vi "Lidar Parsing.vi"() -> ()   [LabVIEW 2016]
uses:
  <vilib>/Platform/TimedLoop/XDataNode/timing_clust.ctl
  <vilib>/Platform/TimedLoop/XDataNode/nitl_modes.ctl
  <vilib>/Platform/TimedLoop/XDataNode/wakeup.ctl
  <vilib>/Platform/TimedLoop/XDataNode/XDataNode.xnode
  <vilib>/Platform/TimedLoop/XDataNode/XDNodeRunTimeDep.lvlib
panel:
  out "쉬프트":cluster{dbl[], dbl[]}(graph)
  in  "쉬프트(mm)":dbl=420.0
  in  "Angular resolution 0.25 / 0.5":dbl=0.25
  in  "finish angle":dbl=180.0
  in  "start angle":dbl
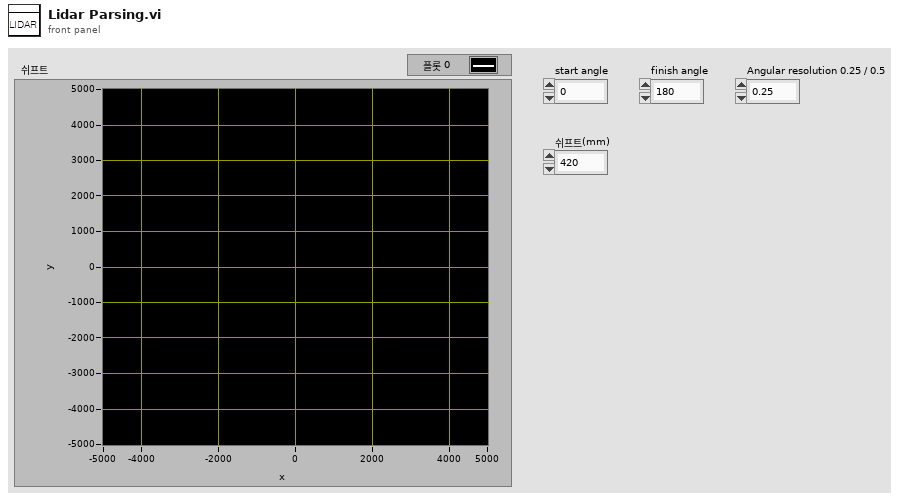
[diagram p1: front panel]
types:
  T1 = enum16{"Standard", "Buffered", "CRLF", "Immediate"}
  T2 = typedef "XDNodeRunTimeDep.lvlib/timing_clust.ctl" = cluster{"Expected End [f-1]":u64, "Actual End [f-1]":u64, "Finished Late? [f-1]":bool, "Expected End [i-1]":u64, "Actual End [i-1]":u64, "Finished Late? [i-1]":bool, "Expected Start [i]":u64, "Actual Start [i]":u64, "Expected Start [f]":u64, "Actual Start [f]":u64, "Source Name":string, "Structure Name":string, "Period":i64, "Deadline":i64, "Offset":i64, "Start":i64, "Priority":i32, "Timeout":i32, "Mode":T3, "Wakeup Reason":T4, "Error":errorcluster, "Source Type":string, "Secondary Source Type":string, "Global End Time":u64, "Global Start Time":u64, "Frame Duration":u64, "Iteration Duration":u64, "Assigned CPU":i32, "I/O Scan Engine Mode":u32}
  T3 = typedef "XDNodeRunTimeDep.lvlib/nitl_modes.ctl" = enum32{"No Change", "Process missed periods, maintain original phase", "Discard missed periods, maintain original phase", "Process missed periods, ignore original phase", "Discard missed periods, ignore original phase"}
  T4 = typedef "XDNodeRunTimeDep.lvlib/wakeup.ctl" = enum32{"Normal", "Aborted", "Asynchronous wakeup", "Timing source error", "Timed loop error", "Timeout"}
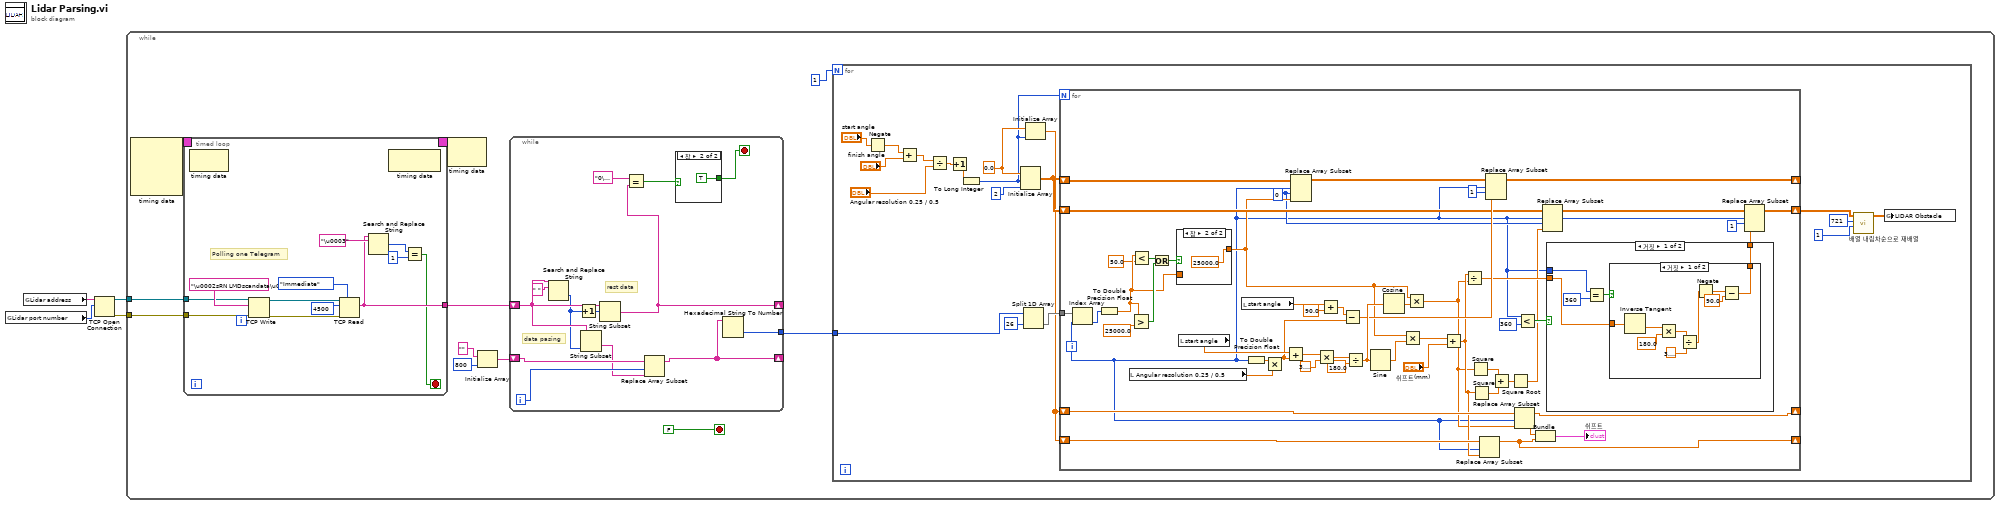
[diagram p0: block diagram]
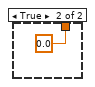
[diagram p2: hidden frame]
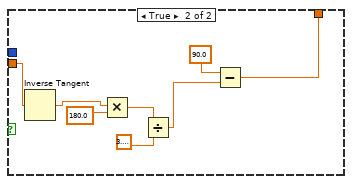
[diagram p3: hidden frame]
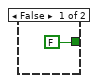
[diagram p5: hidden frame]
diagram:
  n1 = global read "[GV]_LIDAR Port NUM.vi" "Lidar port number"() -> (w1:u16)
  n2 = global read "[GV]_LIDAR Ethernet Address.vi" "Lidar address"() -> (w2:string)
  n3 = TCP Open Connection(address=w2, remote port or service name=w1) -> (connection ID=w4:refnum<k5>, error out=w3:errorcluster)  [unwired: 3 in]
  n4 = while {
    tunnel: w4 -> [w14]
    tunnel: w3 -> [w13]
    stop <- FALSE stop-if-true
    n5 = node-c288() -> (w6:T2)  [unwired: 4 in]
    n6 = timed-loop {
      tunnel: w14 -> [w24]
      tunnel: w13 -> [w23]
      tunnel: [w17] -> w12
      timing: w6 -> [_]
      timing-out: [_] -> w5
      stop <- w16 stop-if-true
      # "Polling one Telegram"
      n7 = node-c288() -> ()  [unwired: 1 in, 1 out]
      n8 = TCP Write(connection ID=w24, data in="\u0002sRN LMDscandata\u0003" ("데이터 입력"), error in (no error)=w23) -> (connection ID out=w27:refnum<k5>, error out=w26:errorcluster)  [unwired: 1 in, 1 out]
      n9 = TCP Read(connection ID=w27, bytes to read=4500 ("읽을 바이트"), error in (no error)=w26, 7:T1."Immediate" ("모드(standard)")) -> (data out=w17:string)  [unwired: 1 in, 2 out]
      n10 = Search and Replace String(input string=w17, search string="\u0003" ("데이터 입력")) -> (number of replacements=w19:i32)  [unwired: 6 in, 3 out]
      n11 = node-c288() -> ()  [unwired: 1 in, 1 out]
      n12 = Equal?(x=w19, y=1) -> (x = y?=w16:bool)
    }
    n13 = node-c288(w5) -> ()  [unwired: 1 out]
    n14 = Initialize Array("", 800 ("차원 크기")) -> (w11:string[])
    n15 = while {
      shift-right: [w132] -> _
      shift-left: w12 -> [w138]
      shift-right: [w129] -> _
      shift-left: w11 -> [w135]
      tunnel: [w128] -> w8
      i -> [w134]
      stop <- w130 stop-if-true
      # "data pasing"
      # "rest data"
      n16 = Search and Replace String(input string=w138, search string=" " ("검색 문자열")) -> (offset past replacement=w137:i32)  [unwired: 6 in, 3 out]
      n17 = Increment(x=w137) -> (x+1=w136:i32)
      n18 = String Subset(string=w138, length (rest)=w137) -> (substring=w133:string)  [unwired: 1 in]
      n19 = String Subset(string=w138, offset (0)=w136) -> (substring=w132:string)  [unwired: 1 in]
      n20 = Equal?(x="0\u0003" ("데이터 입력"), y=w132) -> (x = y?=w131:bool)
      n21 = Replace Array Subset(array=w135, new element=w133, index=w134) -> (w129:string[])
      n22 = case shown="참" w131 {
        tunnel: [FALSE TRUE] -> w130
        frame False {
        }
        frame True {
        }
      }
      n23 = Hexadecimal String To Number(string=w129) -> (number=w128:u32[])  [unwired: 2 in, 1 out]
    }
    n24 = for {
      N: 1 -> [_]
      tunnel: w8 -> [w50]
      w35 = 0.0 ("원소")
      n25 = Negate(x="start angle") -> (-x=w45:dbl)
      n26 = Add(x=w45, y="finish angle") -> (x+y=w42:dbl)
      n27 = Divide(x=w42, y="Angular resolution 0.25 / 0.5") -> (x/y=w46:dbl)
      n28 = Increment(x=w46) -> (x+1=w41:dbl)
      n29 = To Long Integer(number=w41) -> (32bit integer=w34:i32)
      n30 = Initialize Array(w35, w34, 2 ("차원 크기")) -> (w39:dbl[][])
      n31 = Split 1D Array(array=w50, index=26 ("인덱스")) -> (second subarray=w48:u32[])  [unwired: 1 out]
      n32 = Initialize Array(w35, w34) -> (w33:dbl[])
      n33 = for {
        N: w34 -> [_]
        tunnel: w48 -> [w101]
        shift-right: [w77] -> _
        shift-left: w39 -> [w85]
        shift-right: [w62] -> w36
        shift-left: w39 -> [w69]
        shift-right: [w52] -> _
        shift-left: w33 -> [w57]
        shift-right: [w51] -> _
        shift-left: w33 -> [w56]
        i -> [w53]
        w61 = 0 ("비활성화된 인덱스 (열)")
        n34 = Index Array(array=w101, index=w53) -> (element=w92:u32)
        n35 = To Double Precision Float(number=w92) -> (double precision float=w74:dbl)
        n36 = local read "Angular resolution 0.25 / 0.5"() -> (w99:dbl)
        n37 = Greater?(x=w74, y=25000.0) -> (0:w87:bool)
        n38 = Less?(x=w74, y=50.0 ("x")) -> (x < y?=w88:bool)
        n39 = Or(x=w88, y=w87) -> (x .or. y?=w86:bool)
        n40 = case shown="참" w86 {
          tunnel: w74 -> [w125 _]
          tunnel: [w125 25000.0 ("y")] -> w66
          frame False {
          }
          frame True {
          }
        }
        n41 = local read "start angle"() -> (w100:dbl)
        n42 = local read "start angle"() -> (w80:dbl)
        n43 = To Double Precision Float(number=w53) -> (double precision float=w98:dbl)
        n44 = Multiply(x=w98, y=w99) -> (x*y=w82:dbl)
        n45 = Add(x=w100, y=w82) -> (x+y=w96:dbl)
        n46 = Replace Array Subset(array=w85, new element=w66, index (row)=w53, index (col)=w61) -> (w84:dbl[][])
        n47 = Multiply(x=w96, y=3.141592653589793) -> (x*y=w94:dbl)
        n48 = Add(x=w80, y=90.0 ("x")) -> (x+y=w79:dbl)
        n49 = Subtract(x=w79, y=w82) -> (x-y=w78:dbl)
        n50 = Divide(x=w94, y=180.0) -> (x/y=w93:dbl)
        n51 = Sine(x=w93) -> (sin(x)=w90:dbl)
        n52 = Cosine(x=w93) -> (cos(x)=w91:dbl)
        n53 = Multiply(x=w66, y=w90) -> (x*y=w76:dbl)
        n54 = Multiply(x=w66, y=w91) -> (x*y=w54:dbl)
        n55 = Add(x=w76, y="쉬프트(mm)") -> (x+y=w55:dbl)
        n56 = Divide(x=w55, y=w54) -> (x/y=w65:dbl)
        n57 = Square(x=w54) -> (x^2=w72:dbl)
        n58 = Square(x=w55) -> (x^2=w71:dbl)
        n59 = Replace Array Subset(array=w56, new element=w55, index=w53) -> (w51:dbl[])
        n60 = Replace Array Subset(array=w84, new element=w78, index (row)=w53, index (col)=1 ("비활성화된 인덱스 (열)")) -> (w77:dbl[][])
        n61 = Add(x=w72, y=w71) -> (x+y=w70:dbl)
        n62 = Square Root(x=w70) -> (sqrt(x)=w59:dbl)
        n63 = Replace Array Subset(array=w57, new element=w54, index=w53) -> (w52:dbl[])
        n64 = Less?(x=w53, y=360) -> (x < y?=w63:bool)
        n65 = Bundle(w52, w51) -> (→"쉬프트":cluster{dbl[], dbl[]})  [unwired: 1 in]
        n66 = Replace Array Subset(array=w69, new element=w59, index (row)=w53, index (col)=w61) -> (w67:dbl[][])
        n67 = case shown="거짓" w63 {
          tunnel: w65 -> [w103 w124]
          tunnel: w53 -> [w104 _]
          tunnel: [w102 w117] -> w60
          frame False {
            n68 = Equal?(x=w104, y=360) -> (x = y?=w106:bool)
            n69 = case shown="거짓" w106 {
              tunnel: [w107 0.0] -> w102
              tunnel: w103 -> [w111 _]
              frame False {
                n70 = Inverse Tangent(1:w111) -> (0:w112:dbl)
                n71 = Multiply(x=w112, y=180.0) -> (x*y=w114:dbl)
                n72 = Divide(x=w114, y=3.141592653589793) -> (x/y=w110:dbl)
                n73 = Negate(x=w110) -> (-x=w109:dbl)
                n74 = Subtract(x=w109, y=90.0) -> (x-y=w107:dbl)
              }
              frame True {
              }
            }
          }
          frame True {
            n75 = Inverse Tangent(1:w124) -> (0:w118:dbl)
            n76 = Multiply(x=w118, y=180.0) -> (x*y=w120:dbl)
            n77 = Divide(x=w120, y=3.141592653589793) -> (x/y=w123:dbl)
            n78 = Subtract(x=90.0, y=w123) -> (x-y=w117:dbl)
          }
        }
        n79 = Replace Array Subset(array=w67, new element=w60, index (row)=w53, index (col)=1 ("비활성화된 인덱스 (열)")) -> (w62:dbl[][])
      }
      n80 = call "배열 내림차순으로 재배열.vi"("내림차순 기준 인덱스"=1 ("인덱스"), "행 수"=721, "입력 배열"=w36) -> ("출력 배열"=w32:dbl[][])  [unwired: 8 in]
      n81 = global write "[GV]_Lidar Obstacle.vi" "LIDAR Obstacle"(w32) -> ()
    }
  }
